vi "Mouse Move.vi"(7 "Map Model in":refnum<class "Map Model.lvclass">, 8 "error in (no error)":errorcluster, 10 "Position":T1, 11 "Tool in":refnum<class "Tool.lvclass">) -> (0 "error out":errorcluster, 3 "Tool out":refnum<class "Tool.lvclass">, 5 "Map Model out":refnum<class "Map Model.lvclass">)   [LabVIEW 2020, in "Map Model.lvlib" / "Tool.lvclass"]
uses:
  Tool.lvclass
  <vilib>/Utility/miscctls.llb/LVPoint32TypeDef.ctl
  Map Model/Map Model.lvclass
  Tool.lvclass/Tool.ctl
panel:
  # "NOTICE -- YOU MUST LEAVE THIS NOTICE IN PLACE.\n\nCopyright (c) 2017, LIANG LIU Shawn.Liu.cn@gmail.com\nAll rights reserved.\n\nRedistribution and use in source and binary forms, with or without modification, are permitted provided that the following conditions are met:\n-Redistributions of source code must retain the above copyright notice, this list of conditions and the following disclaimer.\n-Redistributions in binary form must reproduce the above copyright notice, this list of conditions and the following disclaimer in the documentation and/or other materials provided with the distribution.\n-Neither the name of the eLp nor the names of its contributors may be used to endorse or promote products derived from this software without specific prior written permission.\n\nTHIS SOFTWARE IS PROVIDED BY THE COPYRIGHT HOLDERS AND CONTRIBUTORS \"AS IS\" AND ANY EXPRESS OR IMPLIED WARRANTIES, INCLUDING, BUT NOT LIMITED TO, THE IMPLIED WARRANTIES OF MERCHANTABILITY AND FITNESS FOR A PARTICULAR PURPOSE ARE DISCLAIMED. IN NO EVENT SHALL THE COPYRIGHT HOLDER OR CONTRIBUTORS BE LIABLE FOR ANY DIRECT, INDIRECT, INCIDENTAL, SPECIAL, EXEMPLARY, OR CONSEQUENTIAL DAMAGES (INCLUDING, BUT NOT LIMITED TO, PROCUREMENT OF SUBSTITUTE GOODS OR SERVICES; LOSS OF USE, DATA, OR PROFITS; OR BUSINESS INTERRUPTION) HOWEVER CAUSED AND ON ANY THEORY OF LIABILITY, WHETHER IN CONTRACT, STRICT LIABILITY, OR TORT (INCLUDING NEGLIGENCE OR OTHERWISE) ARISING IN ANY WAY OUT OF THE USE OF THIS SOFTWARE, EVEN IF ADVISED OF THE POSSIBILITY OF SUCH DAMAGE."
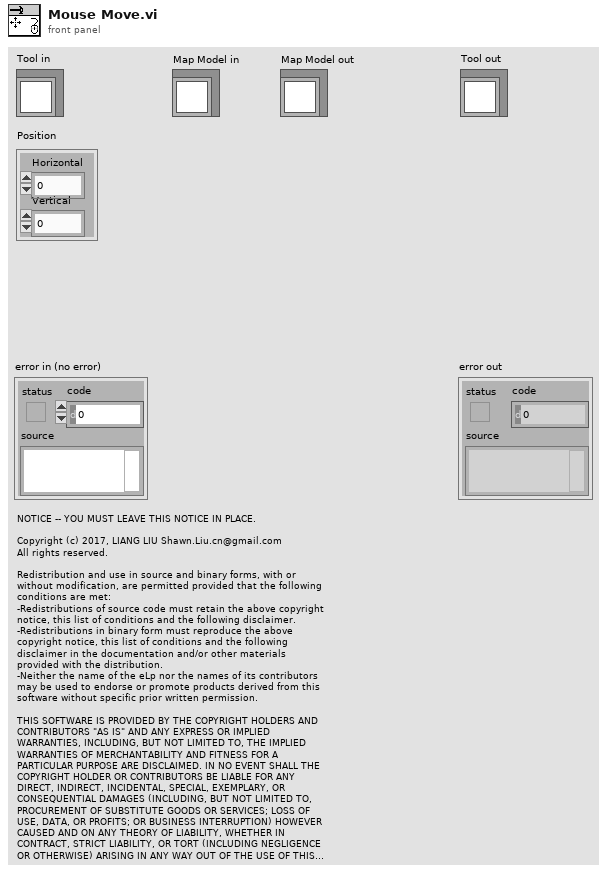
[diagram p1: front panel]
types:
  T1 = typedef "LVPoint32TypeDef.ctl" = cluster{"Horizontal":i32, "Vertical":i32}
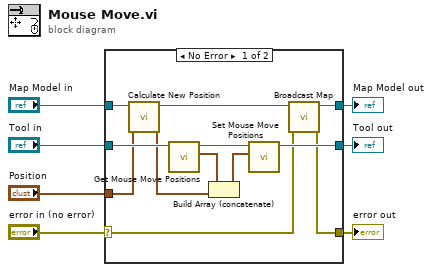
[diagram p0: block diagram]
diagram:
  n1 = case shown="No Error" "error in (no error)" {
    selector: "error in (no error)" -> [w9 w22]
    tunnel: "Tool in" -> [w19 w20]
    tunnel: [w18 w20] -> w6
    tunnel: "Map Model in" -> [w15 w21]
    tunnel: "Position" -> [w12 _]
    tunnel: [w10 w21] -> w3
    tunnel: [w8 w22] -> w1
    frame No Error {
      n2 = call "Calculate New Position.vi"("Position in"=w12, "Map Model in"=w15) -> ("Position out"=w11:T1, "Map Model out"=w14:refnum<class "Map Model.lvclass">)  [unwired: 8 in]
      n3 = call "Get Mouse Move Positions.vi"("Tool in"=w19) -> ("Mouse Move Positions"=w16:T1[], "Tool out"=w17:refnum<class "Tool.lvclass">)  [unwired: 9 in]
      n4 = Build Array (concatenate)(w16, w11) -> (w13:T1[])
      n5 = call "Set Mouse Move Positions.vi"("Mouse Move Positions"=w13, "Tool in"=w17) -> ("Tool out"=w18:refnum<class "Tool.lvclass">)  [unwired: 9 in]
      n6 = call "Broadcast Map.vi"("error in (no error)"=w9, "Map Model in"=w14) -> ("error out"=w8:errorcluster, "Map Model out"=w10:refnum<class "Map Model.lvclass">)  [unwired: 8 in]
    }
    frame Error {
    }
  }
  "error out" <- w1
  "Tool out" <- w6
  "Map Model out" <- w3
